vi "APLUS READ CONFIG.vi"(11 "name or relative path":string="Settings\\Aplus\\Aplus_settings.txt") -> (3 "Array":string[][](array[string]))   [LabVIEW 2019]
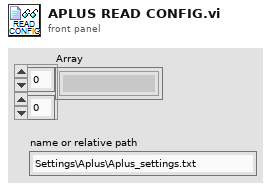
[diagram p1: front panel]
types:
  T1 = enum16{"open", "replace", "create", "open or create", "replace or create", "replace or create with confirmation"}
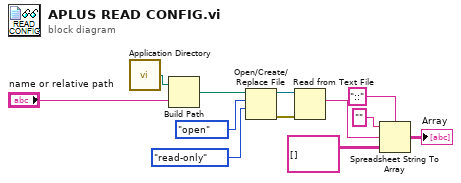
[diagram p0: block diagram]
diagram:
  n1 = call <vilib>:"Application Directory.vi"() -> ("Application Directory"=w1:path)
  n2 = Build Path(base path=w1, name or relative path="name or relative path") -> (appended path=w3:path)
  n3 = Open/Create/Replace File(file path (use dialog)=w3, operation (0:open)=T1."open", access (0:read/write)=enum16{"read/write", "read-only", "write-only"}."read-only") -> (refnum out=w6:refnum<file>, error out=w7:errorcluster)  [unwired: 3 in, 1 out]
  n4 = Read from Text File(file (use dialog)=w6, error in=w7) -> (text=w11:string)  [unwired: 2 in, 3 out]
  n5 = Spreadsheet String To Array(delimiter (Tab)="::", format string="", spreadsheet string=w11, array type (2D Dbl)=string[][] []) -> (array=→"Array":string[][])
